vi "Items To Const.vi"(8 "error in (no error)":errorcluster, 9 "String Item":string, 10 "Multi-Line String":string, 11 "VISA resource name":refnum<visa-resource-name>) -> (0 "error out":errorcluster, 2 "Index":i32, 3 "VISA resource name out":refnum<visa-resource-name>)   [LabVIEW 2013, in "Fluke 5XXX Series Multicalibrators.lvlib"]
doc: "Search for item in array and return index."
uses:
  Fluke 5XXX Series Multicalibrators.lvlib
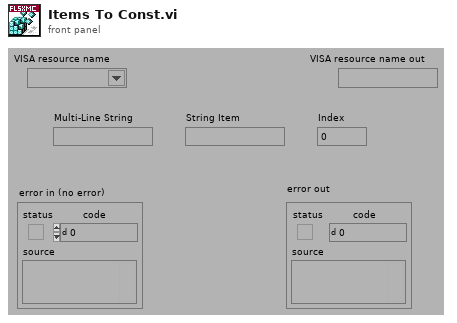
[diagram p1: front panel]
types:
  T1 = cluster{"Status":bool, "Code":i32, "Source (VI Name)":string}
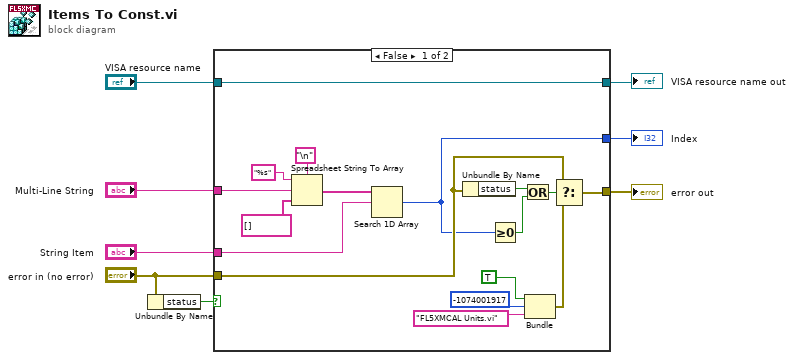
[diagram p0: block diagram]
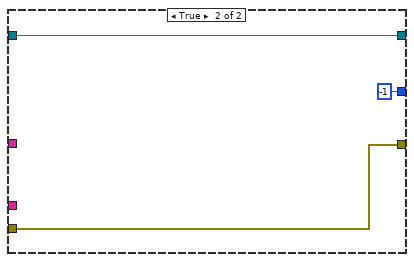
[diagram p2: hidden frame]
diagram:
  n1 = Unbundle By Name("error in (no error)") -> ("status"=w1:bool)
  n2 = case shown="False" w1 {
    tunnel: [w18 w28] -> w8
    tunnel: "error in (no error)" -> [w17 w28]
    tunnel: "Multi-Line String" -> [w13 _]
    tunnel: "String Item" -> [w12 _]
    tunnel: [w10 -1 ("index of element")] -> w5
    tunnel: "VISA resource name" -> [w9 w27]
    tunnel: [w9 w27] -> w3
    frame False {
      n3 = Spreadsheet String To Array(delimiter (Tab)="\n", format string="%s", spreadsheet string=w13, array type (2D Dbl)=string[] [] ("Array Constant")) -> (array=w11:string[])
      n4 = Search 1D Array(1D array=w11, element=w12) -> (index of element=w10:i32)  [unwired: 1 in]
      n5 = Unbundle By Name(w17) -> ("status"=w22:bool)
      n6 = Greater Or Equal To 0?(x=w10) -> (x >= 0?=w24:bool)
      n7 = Or(x=w22, y=w24) -> (x .or. y?=w23:bool)
      n8 = Bundle("Status"=TRUE, "Code"=-1074001917, "Source (VI Name)"="FL5XMCAL Units.vi") -> (w21:T1)  [unwired: 1 in]
      n9 = Select(t=w17, s=w23, f=w21) -> (s? t:f=w18:T1)
    }
    frame True {
    }
  }
  "Index" <- w5
  "error out" <- w8
  "VISA resource name out" <- w3
